vi "Global_SM_Data Out.vi"() -> ()   [LabVIEW 2017, in "LED Signal.lvlib"]
uses:
  LED Signal.lvlib
  Cluster_SM to HW Data.ctl
  <vilib>/Rock Robotics/WPI/SerialPort/WPI_SerialPort.ctl
  ENUM_HW LED Commands.ctl
panel:
  in  "SM LED_HW Cmd Data":T1
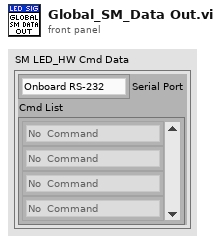
[diagram p1: front panel]
types:
  T1 = typedef "LED Signal.lvlib/Cluster_SM to HW Data.ctl" = cluster{"Serial Port":T2, "Cmd List":T3[]}
  T2 = typedef "WPI_SerialPort.ctl" = enum16{"Onboard RS-232", "MXP TTL", "USB 1", "USB 2"}
  T3 = typedef "LED Signal.lvlib/ENUM_HW LED Commands.ctl" = enum16{"No  Command", "Angled Drive; A", "Field Oriented Drive; D", "Normal Drive; d", "Camera Lined Up; C", "Camera Misallined; c", "Balls in Hopper; B", "Hopper Empty; b"}
diagram:
